vi "Start Impl.vi"(8 "error in (no error)":errorcluster, 11 "Newport Power Meter in":refnum<class "Newport Power Meter.lvclass">) -> (0 "error out":errorcluster, 3 "Newport Power Meter out":refnum<class "Newport Power Meter.lvclass">)   [LabVIEW 2023]
uses:
  Newport Power Meter.lvclass
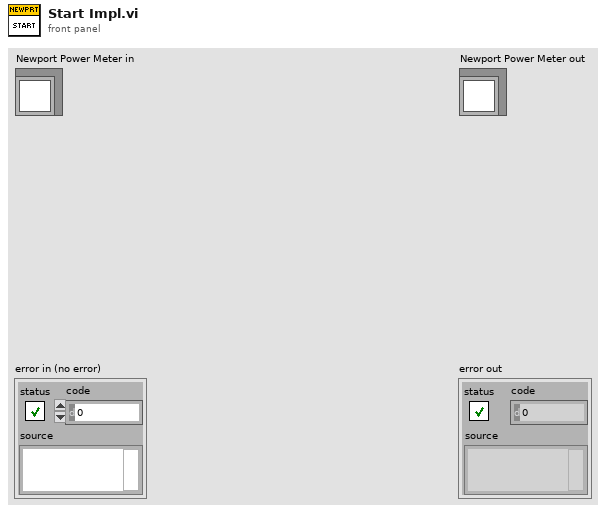
[diagram p1: front panel]
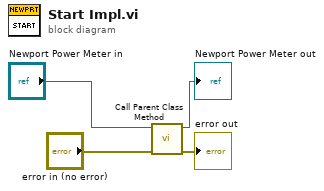
[diagram p0: block diagram]
diagram:
  n1 = call-parent "Call Parent Class Method"("error in (no error)"="error in (no error)", "Power Meter in"="Newport Power Meter in") -> ("error out"=→"error out":errorcluster, "Power Meter out"=→"Newport Power Meter out":refnum<class "Newport Power Meter.lvclass">)  [unwired: 8 in]
